vi "Test_issueCommand_setAuthList.vi"(8 "error in (no error)":errorcluster, 11 "command_setAuthList_Ctl":T1={"TestID"=0, "private_revCode"="        ", "private_sndStamp"=0.0, "private_rcvStamp"=0.0, "private_seqNum"=0, "private_identity"="", "private_origin"=0, "private_host"=0, "authorizedUsers"="", "nonAuthorizedCSCs"=""}) -> (0 "error out":errorcluster, 2 "function return":i32, 3 "command_setAuthList_Ctl out":T1={"TestID"=0, "private_revCode"="        ", "private_sndStamp"=0.0, "private_rcvStamp"=0.0, "private_seqNum"=0, "private_identity"="", "private_origin"=0, "private_host"=0, "authorizedUsers"="", "nonAuthorizedCSCs"=""})   [LabVIEW 2018, in "SALLV_Test.lvlib"]
doc: "int Test_shm_issueCommand_setAuthListLV(Test_command_setAuthListLV *command_setAuthList_Ctl );"
uses:
  DataTypes/command_setAuthList.ctl
  SALLV_Test.lvlib
  SALLV_Test.so
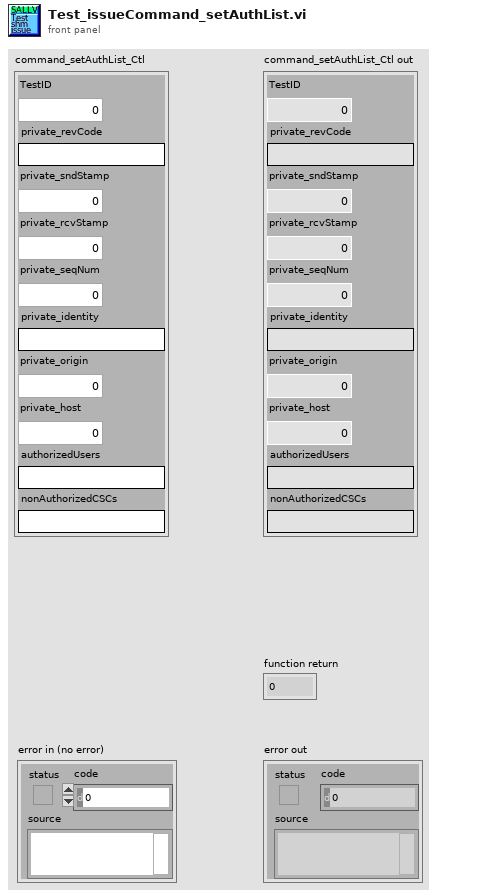
[diagram p1: front panel]
types:
  T1 = typedef "SALLV_Test.lvlib/command_setAuthList.ctl" = cluster{"TestID":i32, "private_revCode":string, "private_sndStamp":dbl, "private_rcvStamp":dbl, "private_seqNum":i32, "private_identity":string, "private_origin":i32, "private_host":i32, "authorizedUsers":string, "nonAuthorizedCSCs":string}
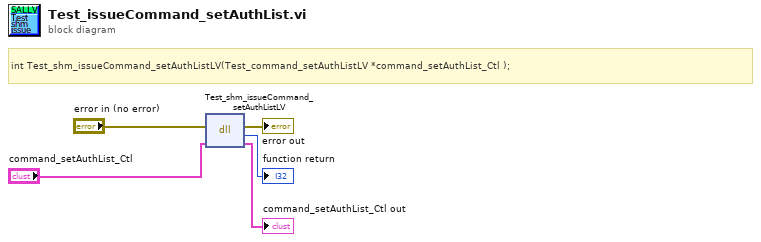
[diagram p0: block diagram]
diagram:
  # "int Test_shm_issueCommand_setAuthListLV(Test_command_setAuthListLV *command_setAuthList_Ctl );"
  n1 = dll-call lib="home/ttsai/Documents/github/ts_SALLabVIEW/testPerfTemp/TestData/SALLV_Test.*" fn="Test_shm_issueCommand_setAuthListLV"(error in="error in (no error)", "command_setAuthList_Ctl"="command_setAuthList_Ctl") -> (error out=→"error out":errorcluster, →"function return":i32, "command_setAuthList_Ctl"=→"command_setAuthList_Ctl out":T1)  [unwired: 2 in, 1 out]
